vi "CleanUp.vi"(0 "object in":refnum<class "Prior_Zmotor.lvclass">, 5 "error in (no error)":errorcluster) -> (14 "object out":refnum<class "Prior_Zmotor.lvclass">, 19 "error out":errorcluster)   [LabVIEW 2021, in "Prior_Zmotor.lvclass"]
uses:
  Prior_Zmotor.lvclass
  Prior_Zmotor.lvclass/Prior_Zmotor.ctl
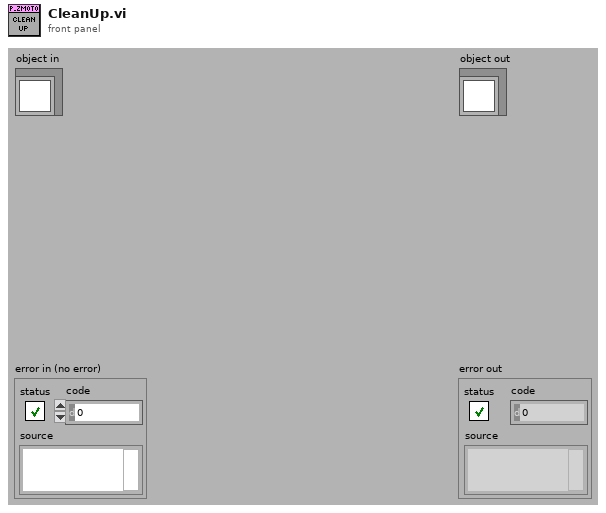
[diagram p1: front panel]
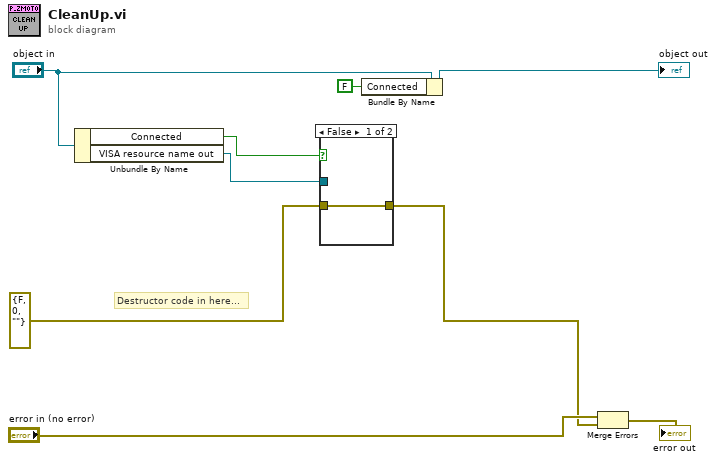
[diagram p0: block diagram]
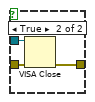
[diagram p2: hidden frame]
diagram:
  # "Destructor code in here..."
  n1 = Unbundle By Name("object in") -> ("Connected"=w1:bool, "VISA resource name out"=w4:refnum<visa-resource-name>)
  n2 = case shown="False" w1 {
    tunnel: w4 -> [_ w13]
    tunnel: errorcluster {"status"=FALSE, "code"=0, "source"=""} ("error in (no error)") -> [w10 w12]
    tunnel: [w10 w11] -> w2
    frame False {
    }
    frame True {
      n3 = VISA Close(VISA resource name=w13, error in (no error)=w12) -> (error out=w11:errorcluster)
    }
  }
  n4 = Bundle By Name(cluster="object in", "Connected"=FALSE) -> (→"object out":refnum<class "Prior_Zmotor.lvclass">)
  n5 = Merge Errors("error in (no error)", w2) -> (→"error out":errorcluster)
